vi "Get GUIDs.vi"(8 "error in (no error)":errorcluster, 11 "Attribute.Dependencies":refnum<class "Attribute.Dependencies.lvclass">) -> (0 "error out":errorcluster, 2 "GUIDs":string[](array[string]), 3 "Variant":variant)   [LabVIEW 2013, in "Attribute.Dependencies.lvclass"]
uses:
  Attribute.Dependencies.lvclass
  Attribute.Dependencies.lvclass/Attribute.Dependencies.ctl
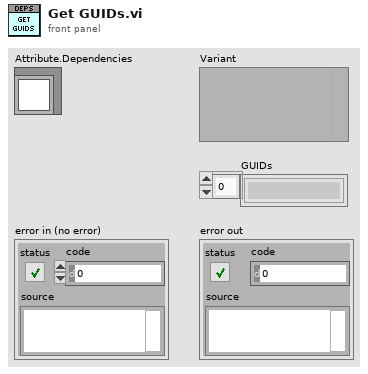
[diagram p1: front panel]
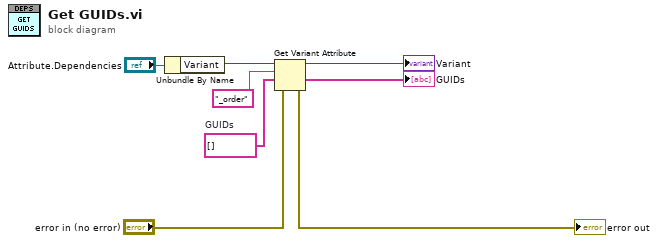
[diagram p0: block diagram]
diagram:
  w4 = string[] []  # GUIDs
  n1 = Unbundle By Name("Attribute.Dependencies") -> ("Variant"=w2:variant)
  n2 = Get Variant Attribute(Variant=w2, name="_order" ("Attribute Name"), default value (empty Variant)=w4, error in="error in (no error)") -> (duplicate Variant=→"Variant":variant, value=→"GUIDs":string[], error out=→"error out":errorcluster)  [unwired: 1 out]
